vi "numchuckDebugger.vi"() -> ()   [LabVIEW 2012]
uses:
  <vilib>/Utility/inputDevices.llb/joystickAcquire.vi
panel:
  in  "device index":i32
  out "Y raw":dbl
  out "X raw":dbl
  in  "deadband":dbl=0.075
  out "button 8":bool
  out "button 6":bool
  out "In Range? Y":bool
  out "In Range? X":bool
  out "Y":dbl
  out "X":dbl
  out "Y":dbl(slide) scale=-1.0..1.0
  out "X":dbl(slide) scale=-1.0..1.0
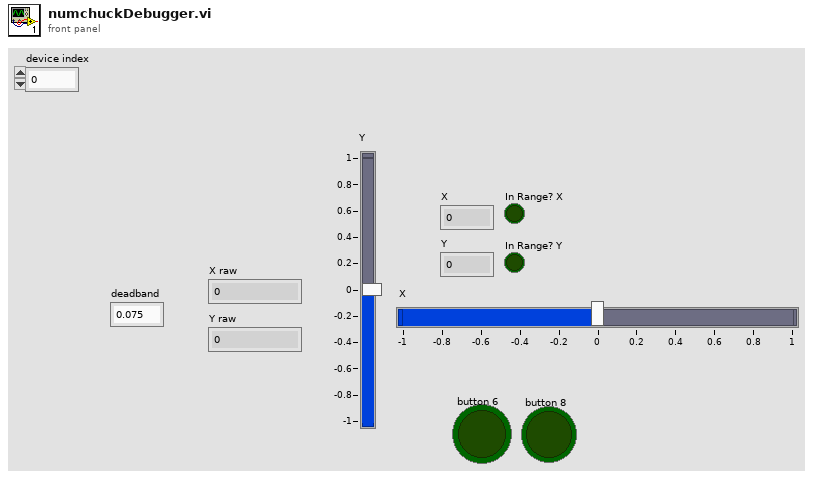
[diagram p1: front panel]
types:
  T1 = cluster{"X axis":dbl, "Y axis":dbl, "Z axis":i32, "X axis rotation":i32, "Y axis rotation":i32, "Z axis rotation":i32, "U axis":i32, "V axis":i32}
  T2 = cluster{"X axis":i32, "Y axis":i32, "Z axis":i32, "X axis rotation":i32, "Y axis rotation":i32, "Z axis rotation":i32, "U axis":i32, "V axis":i32}
  T3 = cluster{"button 1":bool, "button 2":bool, "button 3":bool, "button 4":bool, "button 5":bool, "button 6":bool, "button 7":bool, "button 8":bool, "button 9":bool, "button 10":bool, "button 11":bool, "button 12":bool, "button 13":bool, "button 14":bool, "button 15":bool, "button 16":bool, "button 17":bool, "button 18":bool, "button 19":bool, "button 20":bool, "button 21":bool, "button 22":bool, "button 23":bool, "button 24":bool, "button 25":bool, "button 26":bool, "button 27":bool, "button 28":bool, "button 29":bool, "button 30":bool, "button 31":bool, "button 32":bool}
  T4 = cluster{"X axis":dbl, "Y axis":dbl, "Z axis":dbl, "X axis rotation":dbl, "Y axis rotation":dbl, "Z axis rotation":dbl, "U axis":dbl, "V axis":dbl}
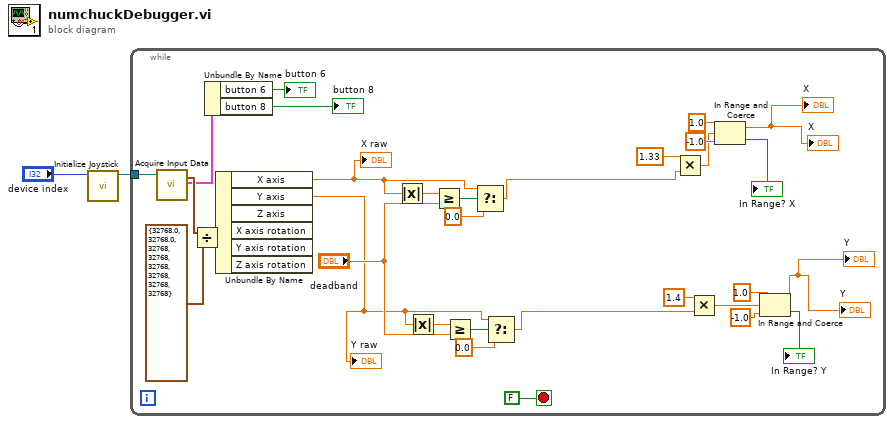
[diagram p0: block diagram]
diagram:
  n1 = call <vilib>:"Initialize Joystick.vi"("device index"="device index") -> ("device ID"=w2:refnum<k1>)  [unwired: 9 in, 1 out]
  n2 = while {
    tunnel: w2 -> [w33]
    stop <- FALSE stop-if-true
    n3 = call-poly <vilib>:"Acquire Input Data.vi"("device ID"=w33) -> ("axis info"=w32:T2, "button info"=w18:T3)  [unwired: 14 in, 3 out]
    n4 = Divide(x=w32, y=T1 {"X axis"=32768.0, "Y axis"=32768.0, "Z axis"=32768, "X axis rotation"=32768, "Y axis rotation"=32768, "Z axis rotation"=32768, "U axis"=32768, "V axis"=32768}) -> (x/y=w29:T4)
    n5 = Unbundle By Name(w18) -> ("button 6"=→"button 6":bool, "button 8"=→"button 8":bool)
    n6 = Unbundle By Name(w29) -> ("X axis"=w5:dbl, "Y axis"=w6:dbl)  [unwired: 4 out]
    "X raw" <- w5
    "Y raw" <- w6
    n7 = Absolute Value(x=w5) -> (abs(x)=w15:dbl)
    n8 = Absolute Value(x=w6) -> (abs(x)=w9:dbl)
    n9 = Greater Or Equal?(x=w15, y="deadband") -> (x >= y?=w14:bool)
    n10 = Greater Or Equal?(x=w9, y="deadband") -> (x >= y?=w10:bool)
    n11 = Select(t=w5, s=w14, f=0.0) -> (s? t:f=w12:dbl)
    n12 = Select(t=w6, s=w10, f=0.0) -> (s? t:f=w7:dbl)
    n13 = Multiply(x=1.33, y=w12) -> (x*y=w24:dbl)
    n14 = Multiply(x=1.4, y=w7) -> (x*y=w21:dbl)
    n15 = In Range and Coerce(upper limit=1.0, x=w24, lower limit=-1.0) -> (coerced(x)=→"X" →"X":dbl, In Range?=→"In Range? X":bool)
    n16 = In Range and Coerce(upper limit=1.0, x=w21, lower limit=-1.0) -> (coerced(x)=→"Y" →"Y":dbl, In Range?=→"In Range? Y":bool)
  }
